vi "Init.vi"(8 "error in (no error)":errorcluster, 11 "Interface VI ref":refnum<vi>) -> (0 "error out":errorcluster)   [LabVIEW 2017, in "WebServiceImporter.lvlib" / "Main Panel.lvlib"]
uses:
  <vilib>/Platform/WebService/Main Panel/Main Panel.lvlib
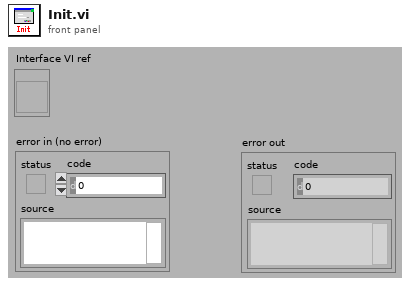
[diagram p1: front panel]
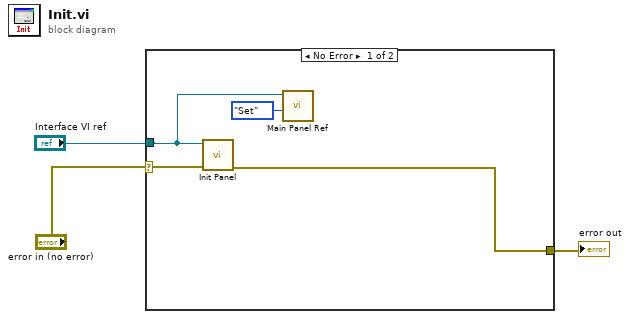
[diagram p0: block diagram]
diagram:
  n1 = case shown="No Error" "error in (no error)" {
    selector: "error in (no error)" -> [w7 w8]
    tunnel: "Interface VI ref" -> [w5 _]
    tunnel: [w4 w8] -> w2
    frame No Error {
      n2 = call <vilib>:"Init Panel.vi"("error in (no error)"=w7, "vi reference"=w5) -> ("error out"=w4:errorcluster)  [unwired: 8 in, 1 out]
      n3 = call <vilib>:"Main Panel Ref.vi"("Operation"=enum16{"Get", "Set"}."Set", "VI Refnum"=w5) -> ()  [unwired: 8 in, 2 out]
    }
    frame Error {
    }
  }
  "error out" <- w2
